vi "未命名 3.vi"() -> ()   [LabVIEW 2018]
panel:
  in  "停止":bool
  out "Image":T1(plugin-control)
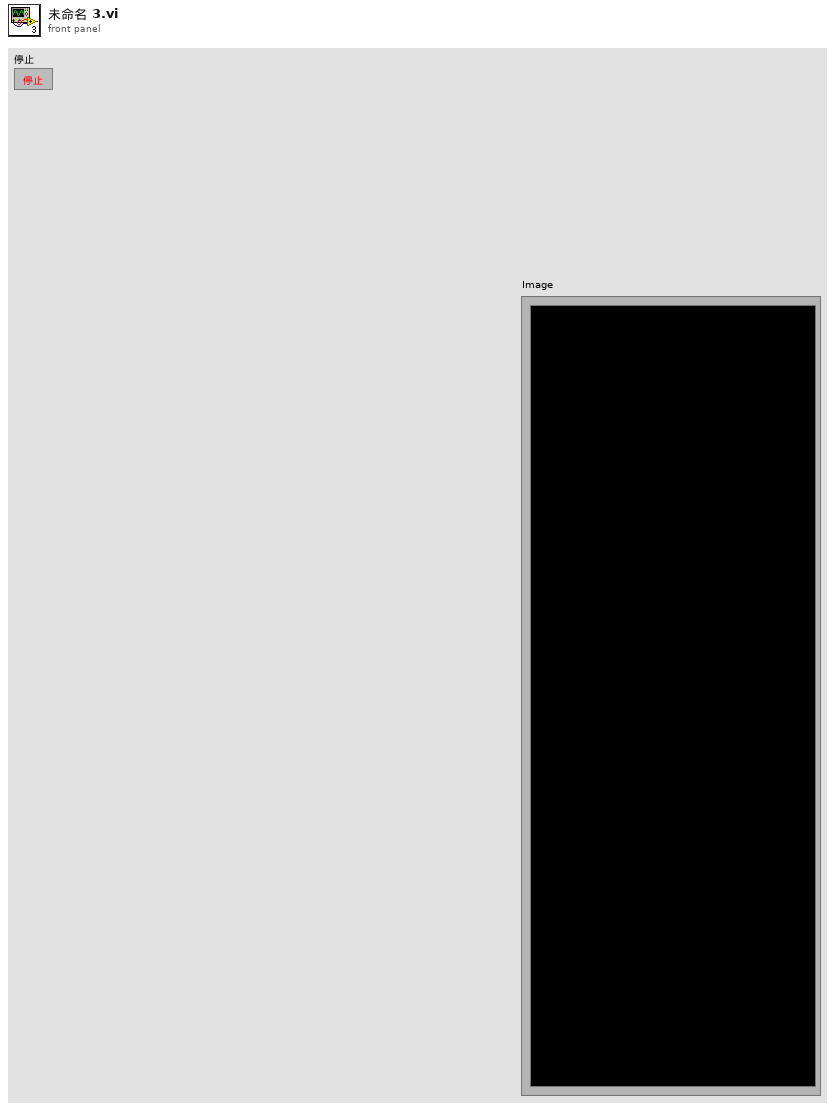
[diagram p1: front panel]
types:
  T1 = typedef "IMAQ Image.ctl" = refnum<image>
  T2 = typedef "Image Type" = u32
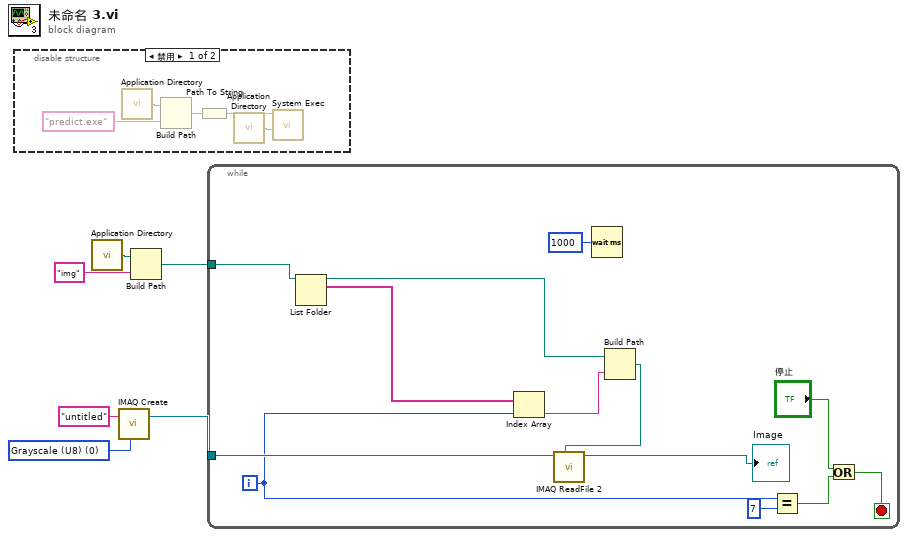
[diagram p0: block diagram]
diagram:
  w2 = T2 0 items=["Grayscale (U8)", "Grayscale (I16)", "Grayscale (SGL)", "Complex (CSG)", "RGB (U32)", "HSL (U32)", "RGB (U64)", "Grayscale (U16)"] ("Image Type")
  n1 = disable-structure shown="禁用" {
    frame Disabled {
      n2 = call <vilib>:"Application Directory.vi"() -> ("Application Directory"=w8:path)
      n3 = Build Path(base path=w8, name or relative path="predict.exe" ("名称或相对路径")) -> (appended path=w10:path)
      n4 = Path To String(path=w10) -> (string=w9:string)
      n5 = call <vilib>:"Application Directory.vi"() -> ("Application Directory"=w11:path)
      n6 = call <vilib>:"System Exec.vi"("working directory"=w11, "command line"=w9) -> ()  [unwired: 6 in, 4 out]
    }
    frame Enabled {
    }
  }
  n7 = call <vilib>:"Application Directory.vi"() -> ("Application Directory"=w5:path)
  n8 = call "IMAQ Create"("Image Name"="untitled", "Image Type"=w2) -> ("New Image"=w1:T1)  [unwired: 3 in, 1 out]
  n9 = Build Path(base path=w5, name or relative path="img" ("名称或相对路径")) -> (appended path=w4:path)
  n10 = while {
    tunnel: w4 -> [w24]
    tunnel: w1 -> [w19]
    i -> [w15]
    stop <- w12 stop-if-true
    n11 = List Folder(path=w24) -> (path out=w22:path, filenames=w23:string[])  [unwired: 3 in, 2 out]
    n12 = Index Array(array=w23, index=w15) -> (element=w21:string)
    n13 = Wait (ms)(milliseconds to wait=u32 1000 ("等待时间（毫秒）")) -> ()  [unwired: 1 out]
    n14 = Build Path(base path=w22, name or relative path=w21) -> (appended path=w20:path)
    n15 = call "IMAQ ReadFile 2"("File Path"=w20, "Image"=w19) -> ("Image Out"=→"Image":T1)  [unwired: 5 in, 4 out]
    n16 = Equal?(x=w15, y=7) -> (x = y?=w13:bool)
    n17 = Or(x="停止", y=w13) -> (x .or. y?=w12:bool)
  }
